vi "数据队列（SGL）.vi"(7 "init":bool caption="初始化", 10 "length":i32=100 caption="采样长度", 11 "input":sgl caption="输入数据点" format="%0.2f") -> (1 "Previous Queue":sgl[](array[numeric]) caption="之前队列", 2 "Current Queue":sgl[](array[numeric]) caption="当前队列", 3 "eliminated":sgl caption="已除去的元素" format="%0.2f", 4 "current length":i32 caption="当前长度")   [LabVIEW 2011]
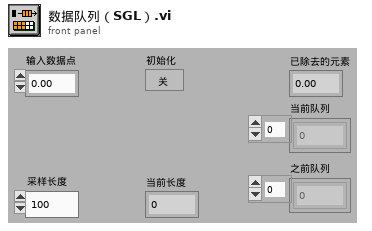
[diagram p1: front panel]
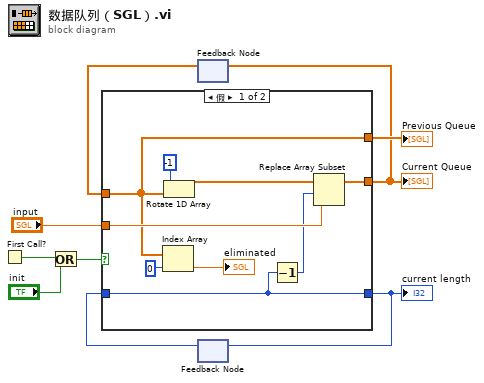
[diagram p0: block diagram]
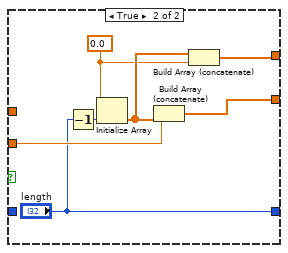
[diagram p2: hidden frame]
diagram:
  n1 = First Call?() -> (First Call?: T/F=w3:bool)
  n2 = Or(x=w3, y="init") -> (x .or. y?=w4:bool)
  n3 = feedback #1() -> (w7:sgl[])  [unwired: 1 in]
  n4 = feedback #2() -> (w8:i32)  [unwired: 1 in]
  n5 = case shown="假" w4 {
    tunnel: [w16 w21] -> w2
    tunnel: [w11 "length"] -> w1
    tunnel: w8 -> [w11 _]
    tunnel: w7 -> [w13 _]
    tunnel: "input" -> [w17 w25]
    tunnel: [w13 w22] -> w9
    frame False {
      n6 = Index Array(array=w13, index=0 ("Index")) -> (element=→"eliminated":sgl)
      n7 = Rotate 1D Array(1:w13, 2:i16 -1 ("n")) -> (0:w14:sgl[])
      n8 = Decrement(x=w11) -> (x-1=w10:i32)
      n9 = Replace Array Subset(array=w14, new element=w17, index=w10) -> (w16:sgl[])
    }
    frame True {
      w19 = sgl 0.0 ("Element Data")
      n10 = Decrement(x="length") -> (x-1=w24:i32)
      n11 = Initialize Array(w19, w24) -> (w23:sgl[])
      n12 = Build Array (concatenate)(w23, w25) -> (w21:sgl[])
      n13 = Build Array (concatenate)(w23, w19) -> (w22:sgl[])
    }
  }
  "Current Queue" <- w2
  "current length" <- w1
  "Previous Queue" <- w9
  n14 = feedback-in #1(w2) -> ()
  n15 = feedback-in #2(w1) -> ()
